vi "Radians to Degrees (Array SGL).vi"(3 "angles (rad)":sgl[](array[numeric])) -> (1 "angles (deg)":sgl[](array[numeric]))   [LabVIEW 2017, in "NI_AngleManipulation.lvlib"]
doc: "Converts a 1D array of angles from radians to degrees."
uses:
  <vilib>/Utility/AngleManip/NI_AngleManipulation.lvlib
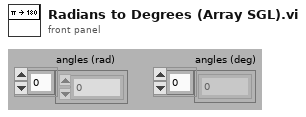
[diagram p1: front panel]
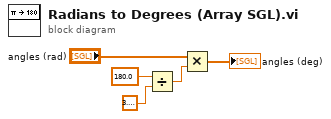
[diagram p0: block diagram]
diagram:
  n1 = Divide(x=sgl 180.0 ("y"), y=sgl 3.1415927) -> (x/y=w3:sgl)
  n2 = Multiply(x="angles (rad)", y=w3) -> (x*y=→"angles (deg)":sgl[])
